vi "VeristandInitialize.vi"(4 "Password":string, 6 "Username":string, 7 "Sequence Context":refnum<k7>, 9 "Visible":bool, 10 "Project File Path":path, 11 "Gateway IP Address (\"\": localhost)":string) -> (0 "error out":errorcluster, 1 "WorkspaceManager out":T1, 2 "Project File Path out":path, 3 "Project Ref out":T2)   [LabVIEW 2015, in "MiscHelperVIs.lvlib"]
uses:
  MiscHelperVIs.lvlib
  <vilib>/NI Veristand/Execution/Project/Project Ref.ctl
  NationalInstruments.VeriStand.ClientAPI
  <vilib>/NI Veristand/Execution/Workspace/WorkspaceAPI.ctl
  <vilib>/NI Veristand/Execution/Project/NI_VS Project ExecutionAPI.lvlib
  <vilib>/NI Veristand/Execution/Workspace/NI_VS Workspace ExecutionAPI.lvlib
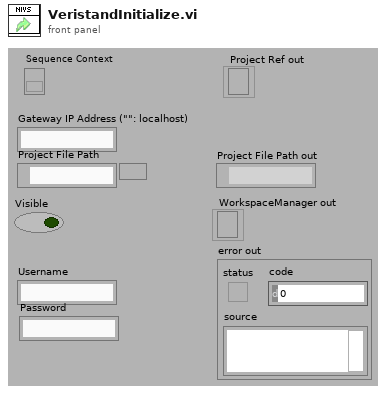
[diagram p1: front panel]
types:
  T1 = typedef "NI_VS Workspace ExecutionAPI.lvlib/WorkspaceAPI.ctl" = refnum<k24>
  T2 = typedef "NI_VS Project ExecutionAPI.lvlib/Project Ref.ctl" = refnum<k24>
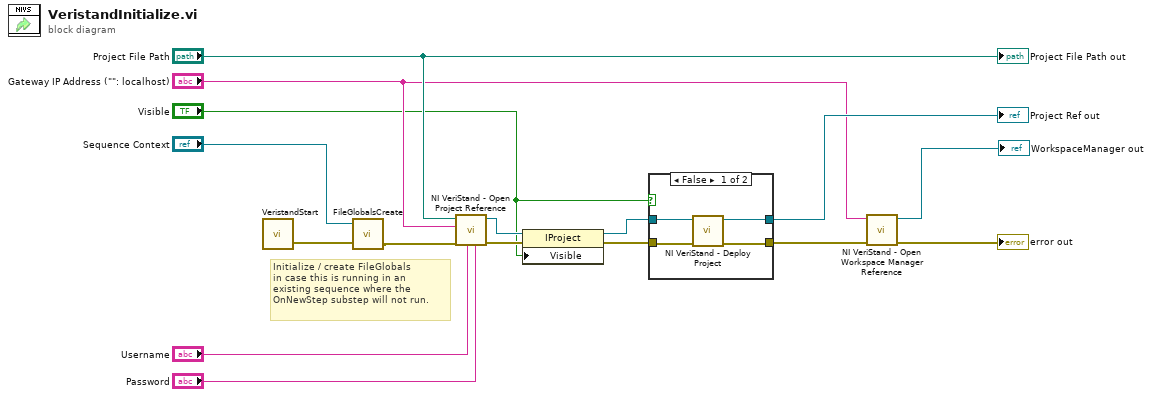
[diagram p0: block diagram]
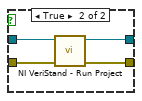
[diagram p2: hidden frame]
diagram:
  # "Initialize / create FileGlobals\nin case this is running in an \nexisting sequence where the \nOnNewStep substep will not run."
  n1 = call "VeristandStart.vi"() -> ("error out"=w10:errorcluster)  [unwired: 3 in]
  n2 = call "FileGlobalsCreate.vi"("error in (no error)"=w10, "Sequence Context"="Sequence Context") -> ("error out"=w9:errorcluster)  [unwired: 3 in]
  n3 = call <vilib>:"NI VeriStand - Open Project Reference.vi"("Password"="Password", "Username"="Username", "error in (no error)"=w9, "Gateway IP Address (\"\": localhost)"="Gateway IP Address (\"\": localhost)", "Project File Path"="Project File Path") -> ("error out"=w13:errorcluster, "Project Ref"=w7:T2)  [unwired: 5 in]
  n4 = property class="IProject"(reference=w7, error in=w13, "Visible"="Visible") -> (reference out=w11:T2, error out=w12:errorcluster)
  n5 = case shown="False" "Visible" {
    tunnel: w12 -> [w20 w24]
    tunnel: w11 -> [w17 w23]
    tunnel: [w18 w22] -> w6
    tunnel: [w19 w21] -> w5
    frame False {
      n6 = call <vilib>:"NI VeriStand - Deploy Project.vi"("error in (no error)"=w20, "Project Ref in"=w17) -> ("error out"=w19:errorcluster, "Project Ref out"=w18:T2)  [unwired: 8 in]
    }
    frame True {
      n7 = call <vilib>:"NI VeriStand - Run Project.vi"("error in (no error)"=w24, "Project Ref in"=w23) -> ("error out"=w21:errorcluster, "Project Ref out"=w22:T2)  [unwired: 8 in]
    }
  }
  "Project Ref out" <- w6
  n8 = call <vilib>:"NI VeriStand - Open Workspace Manager Reference.vi"("error in (no error)"=w5, "Gateway IP Address (\"\": localhost)"="Gateway IP Address (\"\": localhost)") -> ("error out"=→"error out":errorcluster, "WorkspaceManager"=→"WorkspaceManager out":T1)  [unwired: 8 in]
  "Project File Path out" <- "Project File Path"
